vi "Lockin_Amplifier_diag_realtime_optional.vi"(0 "Second":bool, 1 "Sample Number":i32=100000, 2 "all rows":dbl[][](array[numeric]) format="%0.3f", 3 "Cutoff Frequency":dbl=500.0, 4 "dt":dbl=0.0002, 5 "Window (s)":dbl=3.0, 6 "Continous Lock-in":bool, 7 "Resolution":dbl=0.0001, 8 "averaging time":dbl=1.0 format="%0.2p", 9 "Error In":errorcluster, 12 "Sampling Freq":dbl=5000.0, 14 "tolerance (Deviation)":dbl=3.0) -> (13 "Error Out":errorcluster, 15 "dLD_RMS":dbl, 16 "LD_RMS":dbl, 17 "Signal Spectrum":cluster{"f0":dbl, "df":dbl, "magnitude":dbl[]}[](graph), 23 "Time Domain Signal":cluster{"xi used":dbl[], "yi":dbl[]}[](graph), 24 "Phase average":dbl format="%0.2f", 25 "Phase  deviation":dbl format="%0.2f")   [LabVIEW 2013]
uses:
  <vilib>/gmath/NI_Gmath.lvlib
panel:
  in  "DC(V)":dbl
  out "Averaging window":dbl
  in  "Tab Control":T1(tab)
  out "Reference signal / PLL Signal":cluster{"all rows":dbl[], "all rows":dbl[]}[](graph)
  out "Reference Spectrum":cluster{"f0":dbl, "df":dbl, "magnitude":dbl[]}(graph)
  out "Synthetized Spectrum":cluster{"f0":dbl, "df":dbl, "magnitude":dbl[]}(graph)
  in  "t0_ref":dbl
  in  "t0_LD":dbl=0.0001
  out "LD Spectrum":cluster{"f0":dbl, "df":dbl, "magnitude":dbl[]}(graph)
  out "Tolerance Level":dbl
  out "average":dbl
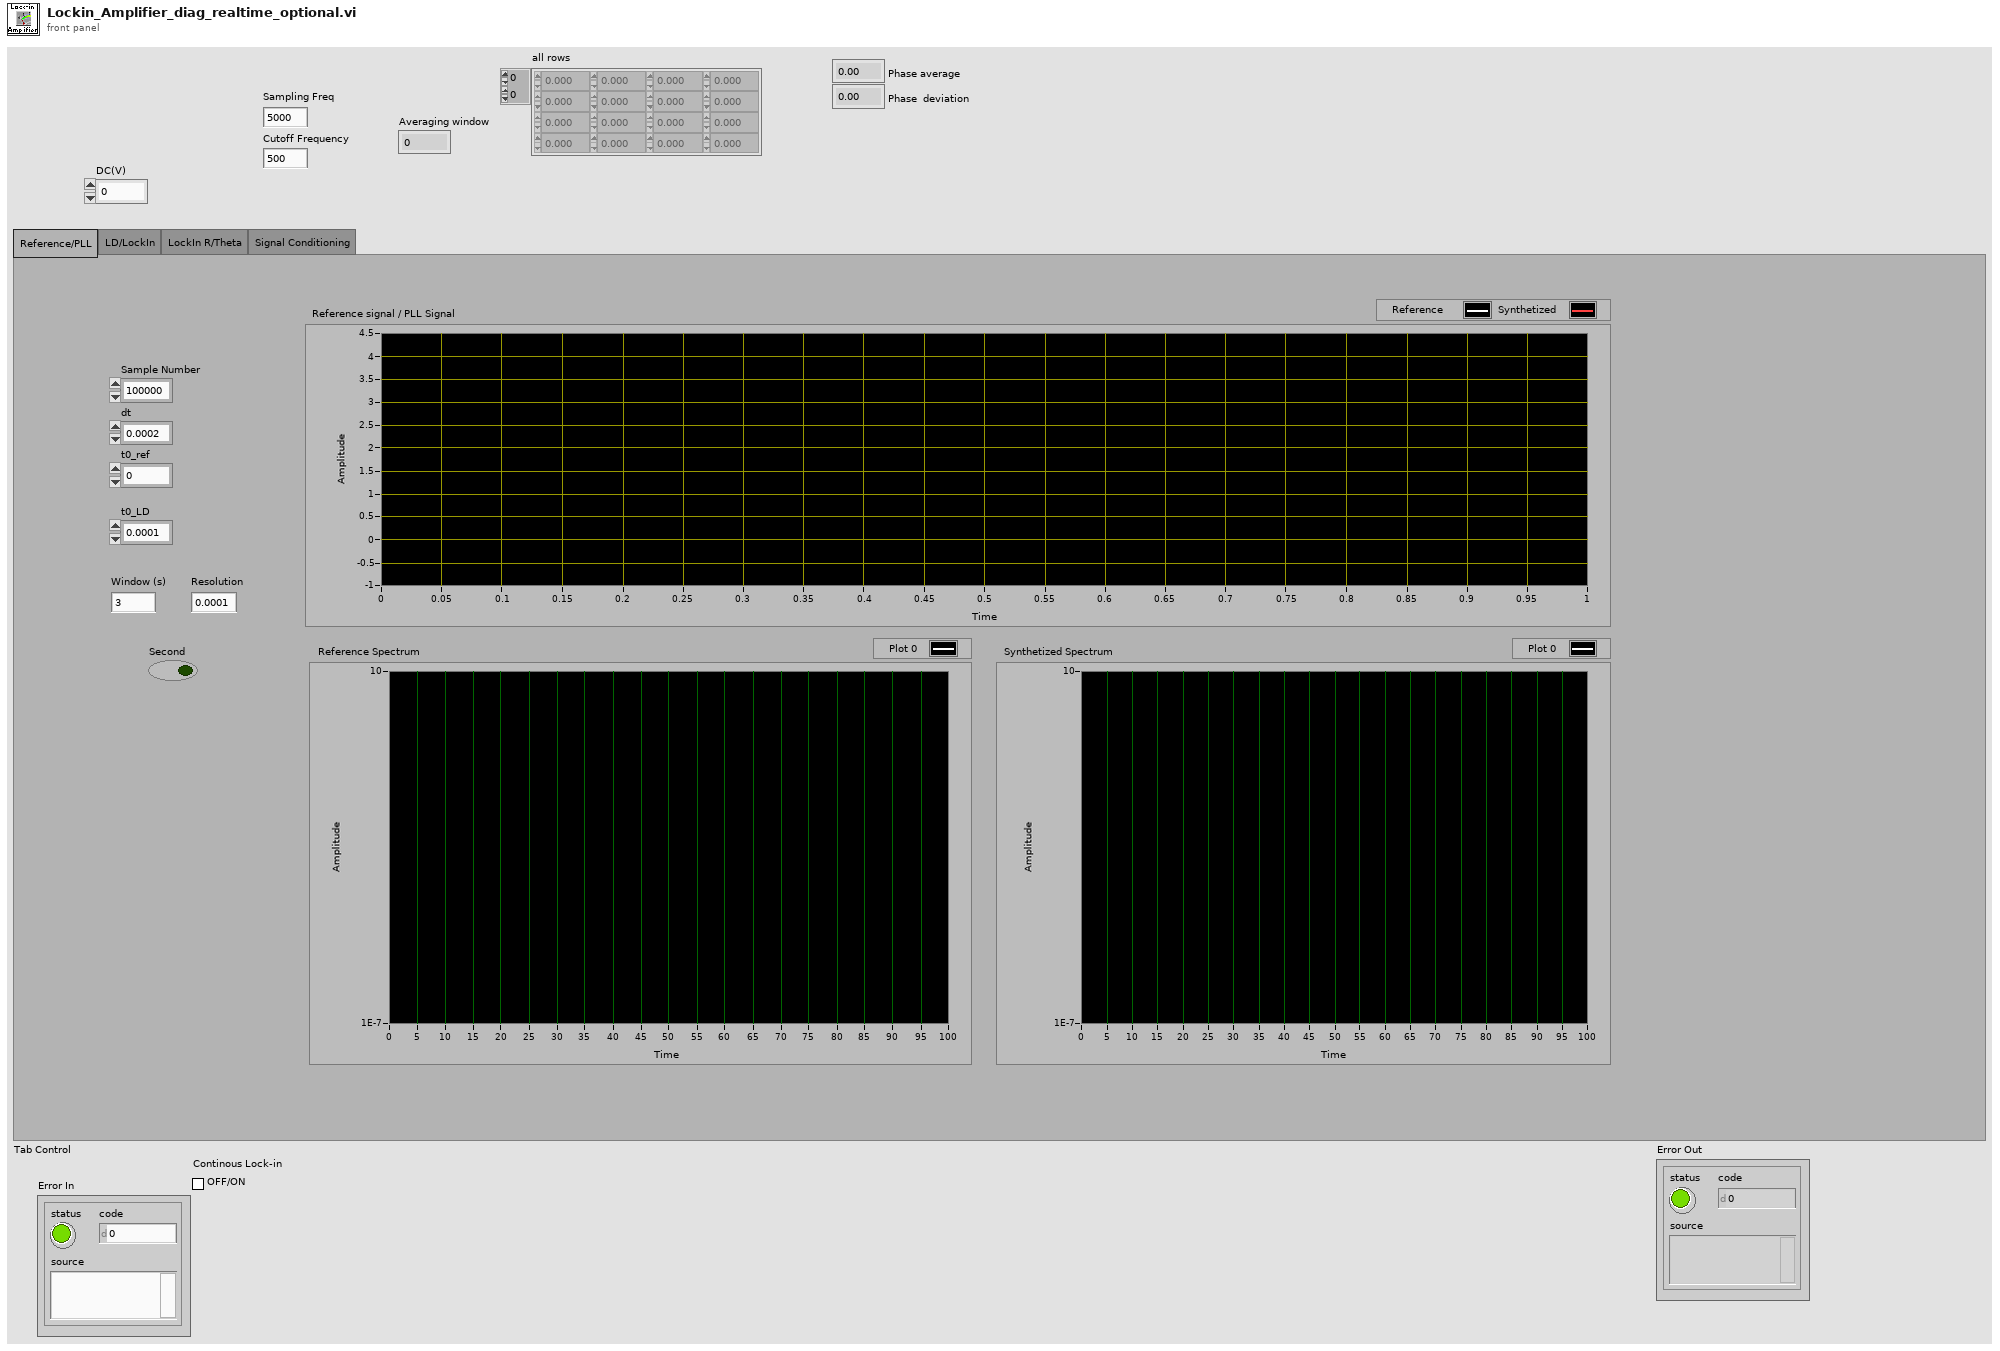
[diagram p1: front panel]
types:
  T1 = enum32{"Reference/PLL", "LD/LockIn", "LockIn R/Theta", "Signal Conditioning"}
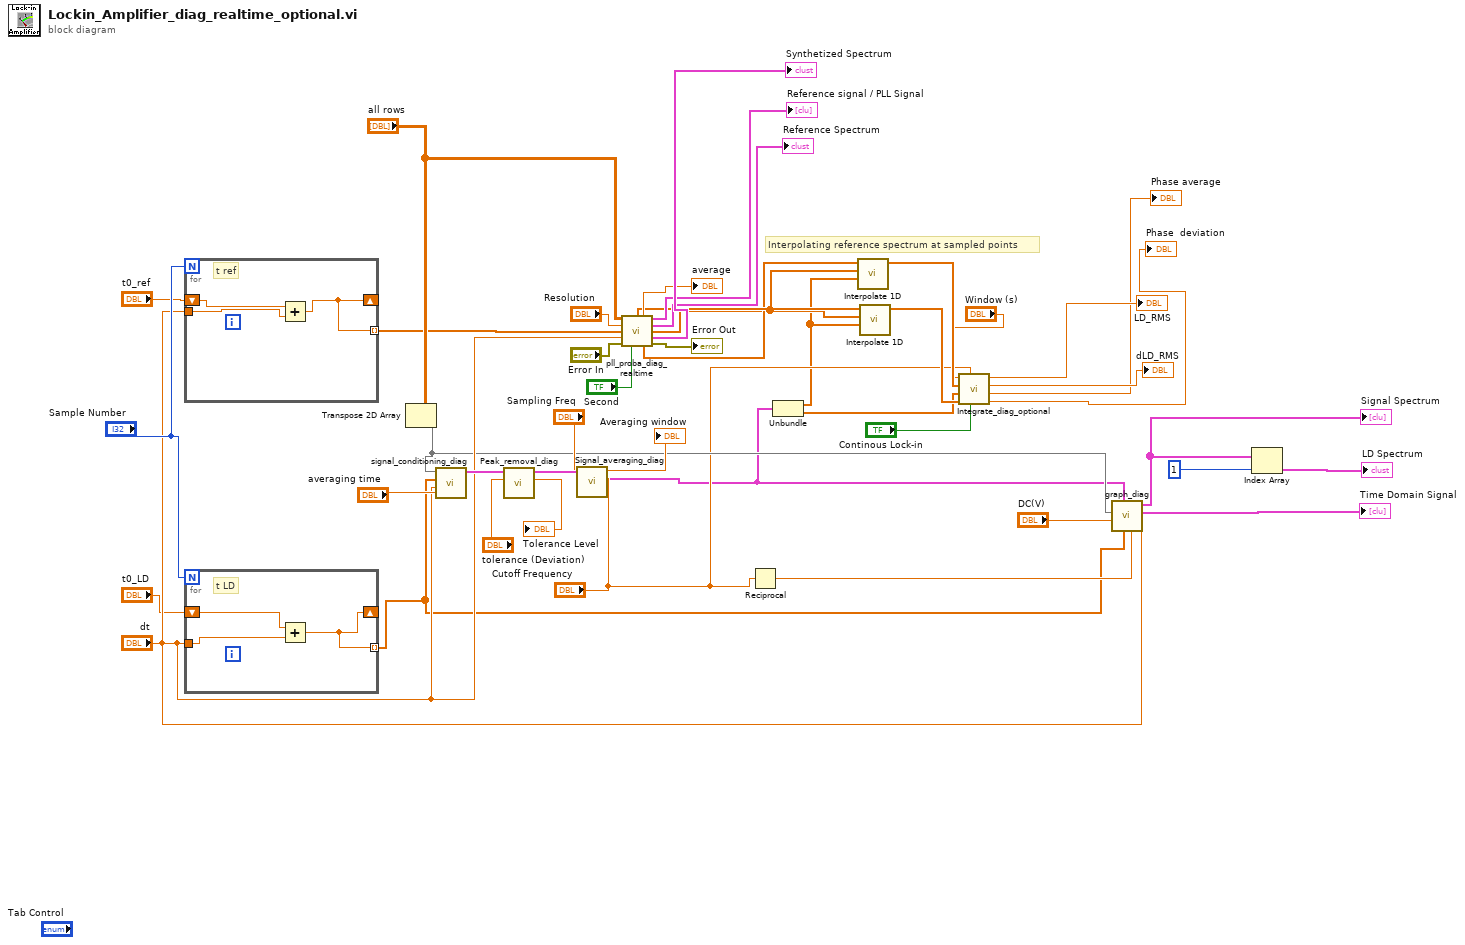
[diagram p0: block diagram]
diagram:
  # "Interpolating reference spectrum at sampled points"
  n1 = for {
    N: "Sample Number" -> [_]
    shift-right: [w45] -> _
    shift-left: "t0_ref" -> [w47]
    tunnel: "dt" -> [w46]
    tunnel: [w45] -> w4 mode=indexing
    # "t ref"
    n2 = Add(x=w47, y=w46) -> (x+y=w45:dbl)
  }
  n3 = for {
    N: "Sample Number" -> [_]
    shift-right: [w48] -> _
    shift-left: "t0_LD" -> [w49]
    tunnel: "dt" -> [w50]
    tunnel: [w48] -> w2 mode=indexing
    # "t LD"
    n4 = Add(x=w49, y=w50) -> (x+y=w48:dbl)
  }
  n5 = Transpose 2D Array(2D array="all rows") -> (transposed array=w20:dbl[][])
  n6 = call "signal_conditioning_diag.vi"("averaging time"="averaging time", "dt"="dt", "t_LD"=w2, "all rows"=w20) -> ("Offset removed"=w32:cluster{"xi used":dbl[], "yi":dbl[]})  [unwired: 6 in, 1 out]
  n7 = call "Peak_removal_diag.vi"("tolerance (Deviation)"="tolerance (Deviation)", "Offset removed"=w32) -> ("Tolerance Level"=→"Tolerance Level":dbl, "XY Graph"=w29:cluster{"xi used":dbl[], "yi":dbl[]})  [unwired: 8 in]
  n8 = call "Signal_averaging_diag.vi"("Pike removed"=w29, "Cutoff Frequency"="Cutoff Frequency", "Sampling Freq"="Sampling Freq") -> ("Averaged"=w8:cluster{"xi used":dbl[], "yi":dbl[]}, "Averaging window"=→"Averaging window":dbl)  [unwired: 7 in]
  n9 = call "pll_proba_diag_realtime.vi"("all rows"="all rows", "Resolution"="Resolution", "t_ref"=w4, "dt"="dt", "Error In"="Error In", "Second"="Second") -> ("average"=→"average":dbl, "XY Graph"=→"Reference signal / PLL Signal":cluster{"all rows":dbl[], "all rows":dbl[]}[], "Waveform Graph"=→"Reference Spectrum":cluster{"f0":dbl, "df":dbl, "magnitude":dbl[]}, "time"=w36:dbl[], "Waveform Graph 2"=→"Synthetized Spectrum":cluster{"f0":dbl, "df":dbl, "magnitude":dbl[]}, "PLL_sine"=w38:dbl[], "PLL_cosine"=w37:dbl[], "Error Out"=→"Error Out":errorcluster)  [unwired: 2 in]
  n10 = Reciprocal(x="Cutoff Frequency") -> (1/x=w10:dbl)
  n11 = Unbundle(w8) -> ("xi used"=w7:dbl[], "yi"=w6:dbl[])
  n12 = call <vilib>:"Interpolate 1D.vi"("xi"=w7, "X"=w36, "Y"=w37) -> ("yi"=w18:dbl[])  [unwired: 6 in, 2 out]
  n13 = call <vilib>:"Interpolate 1D.vi"("xi"=w7, "X"=w36, "Y"=w38) -> ("yi"=w17:dbl[])  [unwired: 6 in, 2 out]
  n14 = call "Integrate_diag_optional.vi"("Continous Lock-in"="Continous Lock-in", "Cutoff Frequency"="Cutoff Frequency", "Ref Sine"=w17, "Processed LD values"=w6, "Ref Cosine"=w18, "Window (s)"="Window (s)") -> ("dTheta"=→"Phase  deviation":dbl, "Theta"=→"Phase average":dbl, "dR"=→"dLD_RMS":dbl, "Lockin R"=→"LD_RMS":dbl)  [unwired: 2 out]
  n15 = call "graph_diag.vi"(4:"dt"=w10, "Array in"=w2, "Averaged"=w8, "DC(V)"="DC(V)", "LD Timetrace in"=w20, 11:"dt"="dt") -> ("Time Domain Signal"=→"Time Domain Signal":cluster{"xi used":dbl[], "yi":dbl[]}[], "Spectra"=w25:cluster{"f0":dbl, "df":dbl, "magnitude":dbl[]}[])  [unwired: 4 in]
  "Signal Spectrum" <- w25
  n16 = Index Array(array=w25, index=1) -> (element=→"LD Spectrum":cluster{"f0":dbl, "df":dbl, "magnitude":dbl[]})
